vi "Edit Goal.vi"(8 "error in (no error)":errorcluster, 9 "Amount":dbl, 10 "Goal ID":i32, 11 "Database in":refnum<class "Database.lvclass">) -> (0 "error out":errorcluster, 3 "Database out":refnum<class "Database.lvclass">)   [LabVIEW 2018, in "Database.lvclass"]
uses:
  Database.lvclass
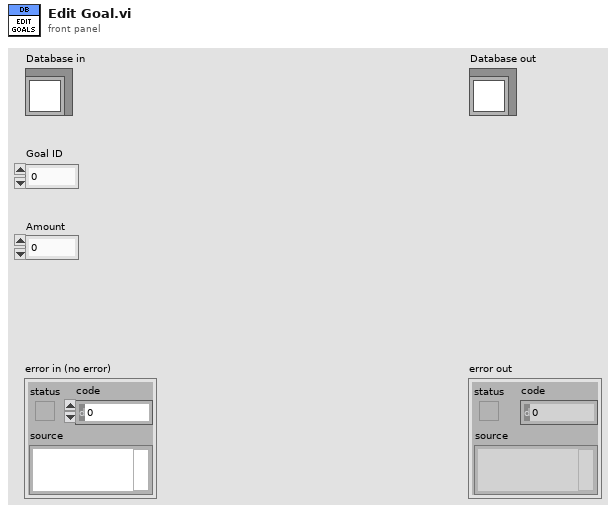
[diagram p1: front panel]
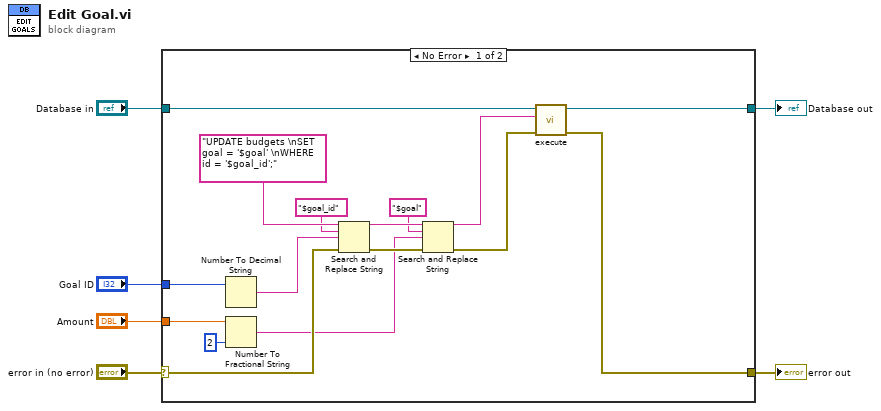
[diagram p0: block diagram]
diagram:
  n1 = case shown="No Error" "error in (no error)" {
    selector: "error in (no error)" -> [w17 w24]
    tunnel: [w20 w24] -> w5
    tunnel: [w21 w23] -> w3
    tunnel: "Database in" -> [w22 w23]
    tunnel: "Goal ID" -> [w13 _]
    tunnel: "Amount" -> [w11 _]
    frame No Error {
      n2 = Number To Decimal String(number=w13) -> (decimal integer string=w12:string)  [unwired: 1 in]
      n3 = Number To Fractional String(number=w11, precision (6)=i16 2) -> (F-format string=w8:string)  [unwired: 2 in]
      n4 = Search and Replace String(input string="UPDATE budgets \nSET goal = '$goal' \nWHERE id = '$goal_id';", search string="$goal_id", replace string=w12, error in=w17) -> (result string=w15:string, error out=w19:errorcluster)  [unwired: 4 in, 2 out]
      n5 = Search and Replace String(input string=w15, search string="$goal", replace string=w8, error in=w19) -> (result string=w14:string, error out=w18:errorcluster)  [unwired: 4 in, 2 out]
      n6 = call "execute.vi"("error in (no error)"=w18, "SQL query"=w14, "Database in"=w22) -> ("error out"=w20:errorcluster, "Database out"=w21:refnum<class "Database.lvclass">)  [unwired: 7 in]
    }
    frame Error {
    }
  }
  "error out" <- w5
  "Database out" <- w3
